vi "Camera Snapshot.vi"() -> ()   [LabVIEW 2014]
doc: "This is the easiest way to capture a frame from a camera."
uses:
  MSC Image_class/MSC Image.lvclass
panel:
  out "error out":errorcluster
  out "picture":picture
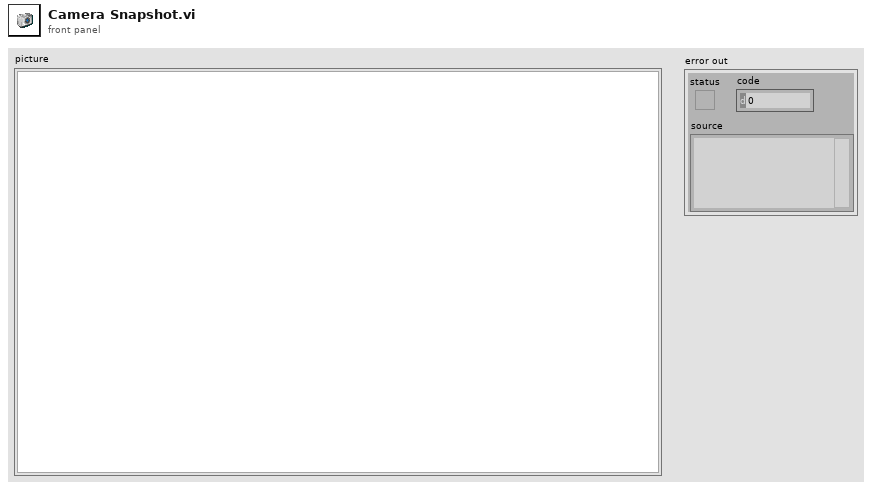
[diagram p1: front panel]
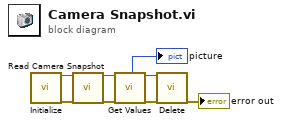
[diagram p0: block diagram]
diagram:
  n1 = call "Initialize.vi"() -> ("image out"=w8:refnum<class "MSC Image.lvclass">, "error out"=w7:errorcluster)  [unwired: 18 in]
  n2 = call-dynamic "Read Camera Snapshot.vi"("image in"=w8, "error in (no error)"=w7) -> ("image out"=w2:refnum<class "MSC Image.lvclass">, "error out"=w1:errorcluster)  [unwired: 16 in]
  n3 = call-dynamic "Get Values.vi"("image in"=w2, "error in (no error)"=w1) -> ("picture"=→"picture":picture, "image out"=w5:refnum<class "MSC Image.lvclass">, "error out"=w3:errorcluster)  [unwired: 10 in, 5 out]
  n4 = call-dynamic "Delete.vi"("image in"=w5, "error in (no error)"=w3) -> ("error out"=→"error out":errorcluster)  [unwired: 17 in]
